vi "Reset green button on multiple.vi"(8 "error in (no error)":errorcluster, 9 "Digital Values":T1[](array[typedef]), 10 "Digital Signal Index":i32, 11 "Controll collection":T2) -> (0 "error out":errorcluster)   [LabVIEW 2011]
uses:
  Controll refrence groups.ctl
  Measurments Handling/Status Digitalish.ctl
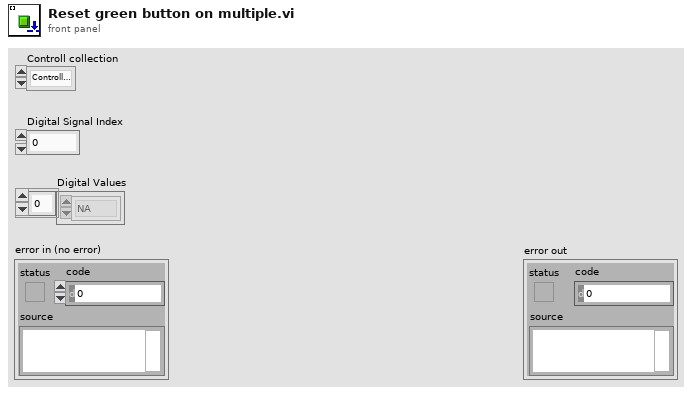
[diagram p1: front panel]
types:
  T1 = typedef "Status Digitalish.ctl" = enum16{"NA", "False", "True"}
  T2 = typedef "Controll refrence groups.ctl" = enum16{"Controller. gen", "Controller . High G", "Stroker", "PCP Online", "PCP Local", "PCP HV On", "Driller", "Stroker Cmd Buttons", "Stroker Anchor Cmd Buttons", "Controller Relay Buttons", "PCP Start Telemetry", "PCP Start Motor", "Tractor", "Modem Status"}
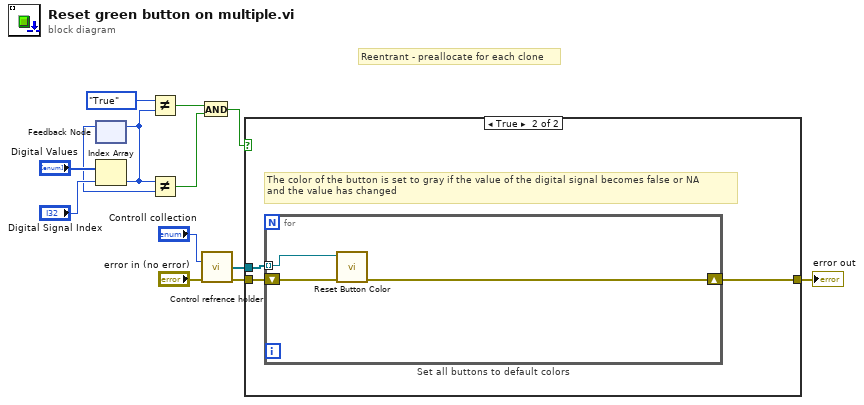
[diagram p0: block diagram]
diagram:
  # "Reentrant - preallocate for each clone"
  n1 = feedback #1() -> (w1:T1)  [unwired: 1 in]
  n2 = Index Array(array="Digital Values", index="Digital Signal Index") -> (element=w2:T1)
  n3 = feedback-in #1(w2) -> ()
  n4 = Not Equal?(x=Status_Digitalish."True", y=w2) -> (x != y?=w7:bool)
  n5 = Not Equal?(x=w2, y=w1) -> (x != y?=w6:bool)
  n6 = And(x=w7, y=w6) -> (x .and. y?=w5:bool)
  n7 = call "Control refrence holder.vi"("Controll collection"="Controll collection", "error in (no error)"="error in (no error)") -> ("Controlls out"=w12:refnum<vi>[], "error out"=w11:errorcluster)  [unwired: 12 in]
  n8 = case shown="True" w5 {
    tunnel: w12 -> [_ w17]
    tunnel: w11 -> [w14 w16]
    tunnel: [w14 w15] -> w9
    frame False {
    }
    frame True {
      # "The color of the button is set to gray if the value of the digital signal becomes false or NA\nand the value has changed"
      n9 = for "Set all buttons to default colors" {
        tunnel: w17 -> [w20] mode=indexing
        shift-right: [w18] -> w15
        shift-left: w16 -> [w19]
        n10 = call "Reset Button Color.vi"("error in (no error)"=w19, "Control in"=w20) -> ("error out"=w18:errorcluster)  [unwired: 9 in]
      }
    }
  }
  "error out" <- w9
